vi "Save All Data.vi"(0 "Config":T1={"DAQ Settings"={"Trigger Type"=enum."Manual", "Trigger Samples"=0, "Pretrigger Samples"=0, "Trigger Interval"=0.0, "Time Units"=FALSE, "Auto Save"=FALSE, "Sample Rate"=7.0, "Select Analog"=FALSE, "Trigger Value"=0.0, "Trigger Stop Method"=enum."Use Samples Value to Stop Trigger", "Rate Sec/Min"=FALSE, "Save Mode"=enum."Single File", "File Size Limit"=0.0, "Log File Type"=enum."Basic", "Trigger Data Index"=0}, "Channels"=[], "Header"={"TA Number"="", "Test Name"="", "Serial Number"="", "Technician"=""}, "Graph Settings"={"Graph Labels"=[], [], [], [], [], [], [], [], [], [], [], [], [], "Graph Toggles"=[], "Axis Toggles"=[], "Graph Range"=enum."1"}, "Test Limits"=[], "All Type Info"=[], "Save Mode"=enum."Single File"} {"DAQ Settings"."Trigger Interval" min=0.0; "DAQ Settings"."Pretrigger Samples" min=0; "DAQ Settings"."Trigger Samples" min=0}, 1 "Sample Rate":sgl, 5 "Data":sgl[][](array[numeric])) -> ()   [LabVIEW 2019]
uses:
  Type Defs and Controls/DAQ Settings.ctl
  Type Defs and Controls/Header.ctl
  Type Defs and Controls/Sensor Config.ctl
  Type Defs and Controls/Channel Config.ctl
  Type Defs and Controls/Trigger Stop Method.ctl
  Type Defs and Controls/Graph Settings Type Def.ctl
  Type Defs and Controls/Log File Type.ctl
  Type Defs and Controls/Test Limits.ctl
  Type Defs and Controls/Part Info.ctl
  Type Defs and Controls/All Part Info.ctl
panel:
  out "transposed array":sgl[][](array[numeric])
  # "EGU"
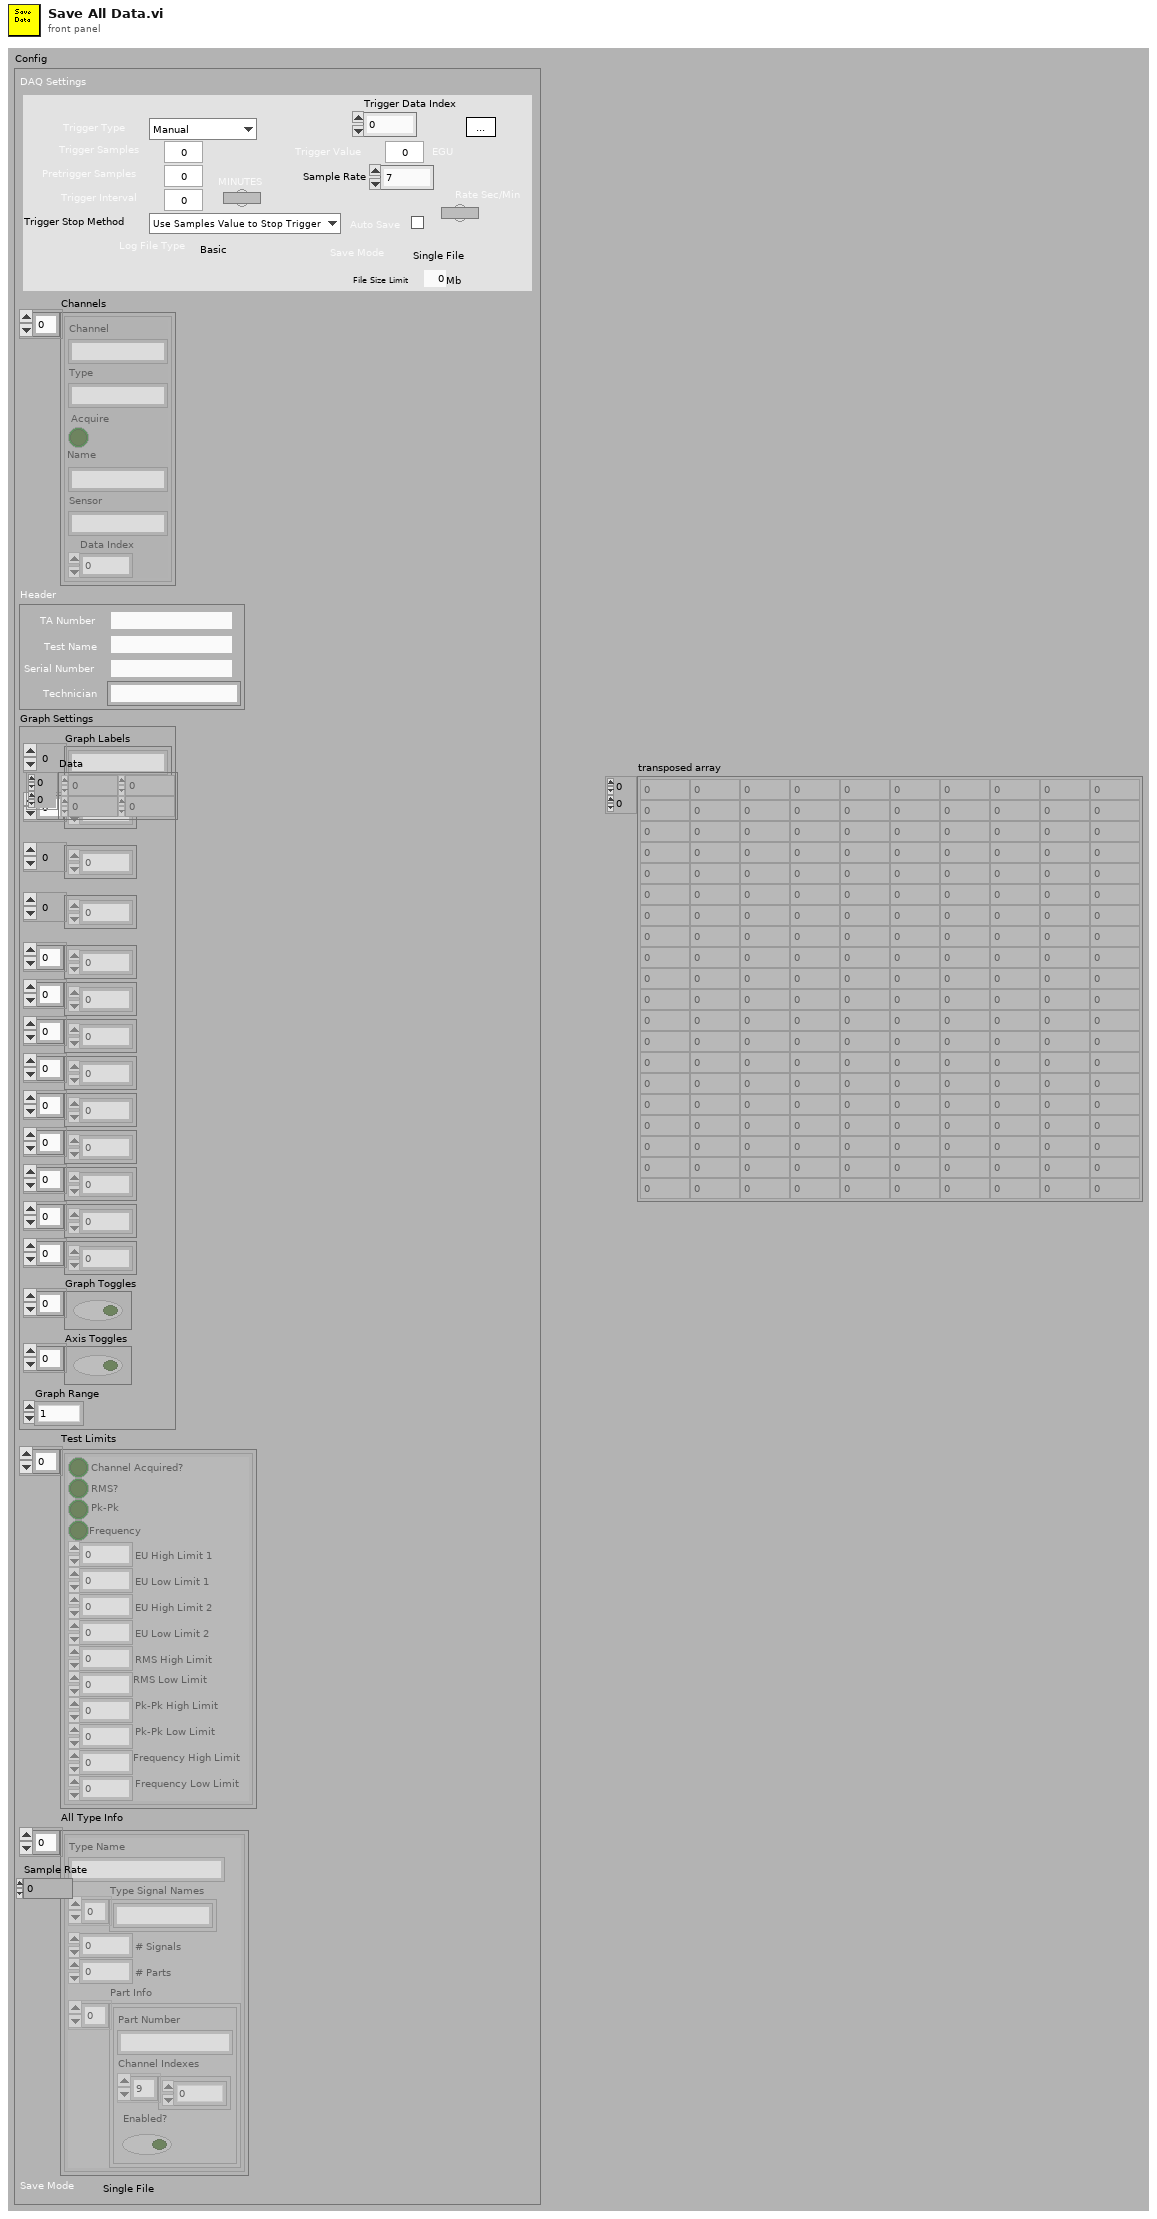
[diagram p1: front panel]
types:
  T1 = typedef "Sensor Config.ctl" = cluster{"DAQ Settings":T2, "Channels":T5[], "Header":T6, "Graph Settings":T7, "Test Limits":T8[], "All Type Info":T9, "Save Mode":enum16{"Single File", "Segmented Files", "New File at Midnight"}}
  T2 = typedef "DAQ Settings.ctl" = cluster{"Trigger Type":enum16{"Manual", "Timed", "Analog Rising", "Analog Falling"}, "Trigger Samples":i32, "Pretrigger Samples":i32, "Trigger Interval":dbl, "Time Units":bool, "Auto Save":bool, "Sample Rate":dbl, "Select Analog":bool, "Trigger Value":dbl, "Trigger Stop Method":T3, "Rate Sec/Min":bool, "Save Mode":enum16{"Single File", "Segmented Files", "New File at Midnight"}, "File Size Limit":dbl, "Log File Type":T4, "Trigger Data Index":u32}
  T3 = typedef "Trigger Stop Method.ctl" = enum16{"Use Samples Value to Stop Trigger", "Use Threshold to Stop Trigger"}
  T4 = typedef "Log File Type.ctl" = enum16{"Basic", "RTS"}
  T5 = typedef "Channel Config.ctl" = cluster{"Channel":string, "Type":string, "Acquire":bool, "Name":string, "Sensor":string, "Data Index":u32}
  T6 = typedef "Header.ctl" = cluster{"TA Number":string, "Test Name":string, "Serial Number":string, "Technician":string}
  T7 = typedef "Graph Settings Type Def.ctl" = cluster{"Graph Labels":string[], u8[], i16[], u32[], u8[], u8[], u8[], u32[], u8[], u8[], u8[], dbl[], dbl[], "Graph Toggles":bool[], "Axis Toggles":bool[], "Graph Range":enum16{"1", "2", "3", "4", "5", "10", "15", "30", "60"}}
  T8 = typedef "Test Limits.ctl" = cluster{"Channel Acquired?":bool, "RMS?":bool, "Pk-Pk":bool, "Frequency":bool, "EU High Limit 1":dbl, "EU Low Limit 1":dbl, "EU High Limit 2":dbl, "EU Low Limit 2":dbl, "RMS High Limit":dbl, "RMS Low Limit":dbl, "Pk-Pk High Limit ":dbl, "Pk-Pk Low Limit":dbl, "Frequency High Limit":dbl, "Frequency Low Limit":dbl}
  T9 = typedef "All Part Info.ctl" = cluster{"Type Name":string, "Type Signal Names":string[], "# Signals":i32, "# Parts":i32, "Part Info":T10[]}[]
  T10 = typedef "Part Info.ctl" = cluster{"Part Number":string, "Channel Indexes":u16[], "Enabled?":bool}
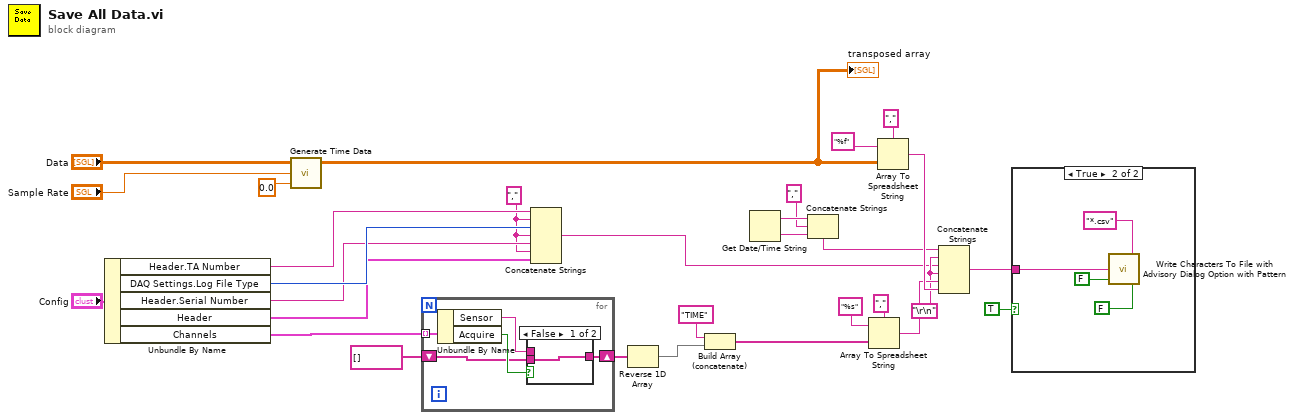
[diagram p0: block diagram]
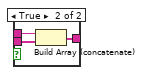
[diagram p3: hidden frame]
diagram:
  w5 = "," ("string")
  w18 = "\r\n"
  n1 = Unbundle By Name("Config") -> ("Header.TA Number"=w9:string, "DAQ Settings.Log File Type"=w8:T4, "Header.Serial Number"=w7:string, "Header"=w6:T6, "Channels"=w29:T5[])
  n2 = call "Generate Time Data.vi"("Time Offset"=sgl 0.0 ("Last Time"), "Sample Rate"="Sample Rate", "Data"="Data") -> ("Array"=w1:sgl[][])  [unwired: 1 in, 1 out]
  "transposed array" <- w1
  n3 = for {
    tunnel: w29 -> [w32] mode=indexing
    shift-right: [w33] -> w21
    shift-left: string[] [] -> [w31]
    n4 = Unbundle By Name(w32) -> ("Sensor"=w34:string, "Acquire"=w35:bool)
    n5 = case shown="False" w35 {
      tunnel: [w36 w39] -> w33
      tunnel: w31 -> [w36 w38]
      tunnel: w34 -> [_ w37]
      frame False {
      }
      frame True {
        n6 = Build Array (concatenate)(w37, w38) -> (w39:string[])
      }
    }
  }
  n7 = Concatenate Strings(w9, w5, w8, w5, w7, w5, w6) -> (w10:string)
  n8 = Reverse 1D Array(array=w21) -> (reversed array=w3:string[])
  n9 = Build Array (concatenate)("TIME", w3) -> (w19:string[])
  n10 = Get Date/Time String() -> (date string=w16:string, time string=w17:string)  [unwired: 3 in]
  n11 = Concatenate Strings(w16, "," ("string"), w17) -> (w15:string)
  n12 = Array To Spreadsheet String(delimiter (Tab)=",", array=w19, 3:"%s" ("format string")) -> (spreadsheet string=w20:string)
  n13 = Array To Spreadsheet String(delimiter (Tab)=",", array=w1, 3:"%f" ("format string")) -> (spreadsheet string=w28:string)
  n14 = Concatenate Strings(w15, w18, w10, w18, w20, w28) -> (w27:string)
  n15 = case shown="True" TRUE ("Case Constant\n(See Context Help)") {
    tunnel: w27 -> [_ w43]
    frame False {
    }
    frame True {
      n16 = call "Write Characters To File with Advisory Dialog Option with Pattern.vi"("advisory dialog? (display:T)"=FALSE, "pattern"="*.csv", "append to file? (new file:F)"=FALSE, "character string"=w43) -> ()  [unwired: 1 in, 1 out]
    }
  }
